vi "Untitled 8.vi"() -> ()   [LabVIEW 2017]
uses:
  control/stateCmdUpdatePara.ctl
  LibraryGcode.lvlib
  control/Queue/QueueCMDandPOS.ctl
  control/Queue/TypeDataPOS.ctl
panel:
  in  "Queue Process":T1
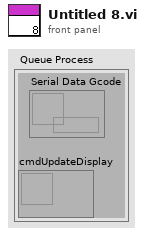
[diagram p1: front panel]
types:
  T1 = typedef "LibraryGcode.lvlib/QueueCMDandPOS.ctl" = cluster{"Serial Data Gcode":refnum<queue>, "cmdUpdateDisplay":refnum<queue>}
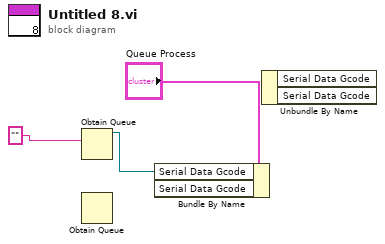
[diagram p0: block diagram]
diagram:
  n1 = Obtain Queue(element data type="") -> (queue out=w3:refnum<queue>)  [unwired: 4 in, 2 out]
  n2 = Obtain Queue() -> ()  [unwired: 5 in, 3 out]
  n3 = Bundle By Name(cluster="Queue Process", "Serial Data Gcode"=w3) -> ()  [unwired: 1 in, 1 out]
  n4 = Unbundle By Name() -> ()  [unwired: 1 in, 2 out]
